vi "SET_SHUNT_n.vi"(2 "execute":bool, 7 "SHUNT values":cdb[](array[numeric]), 11 "error in (no error)":errorcluster) -> (4 "function return":string, 15 "error out":errorcluster)   [LabVIEW 2017, in "ZBOX_IS.lvlib"]
uses:
  ZBOX_IS.lvlib
panel:
  out "BytePtr":u8[](array[numeric])
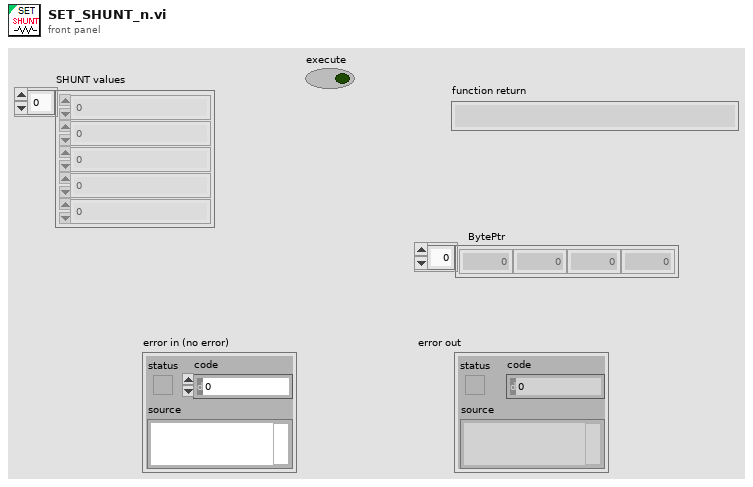
[diagram p1: front panel]
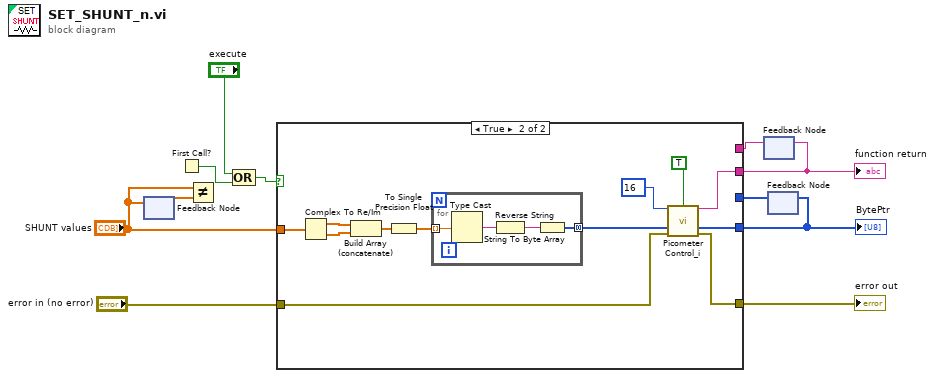
[diagram p0: block diagram]
diagram:
  n1 = feedback-in #1("SHUNT values") -> ()
  n2 = feedback #1() -> (w5:cdb[])  [unwired: 1 in]
  n3 = First Call?() -> (First Call?: T/F=w2:bool)
  n4 = Not Equal?(x="SHUNT values", y=w5) -> ()  [unwired: 1 out]
  n5 = Compound Arithmetic op=OR("execute", w2) -> (w3:bool)
  n6 = feedback #2() -> (w8:string)  [unwired: 1 in]
  n7 = feedback #3() -> (w6:u8[])  [unwired: 1 in]
  n8 = case shown="True" w3 {
    tunnel: "error in (no error)" -> [w14 w25]
    tunnel: [w14 w24] -> w10
    tunnel: [w13 w23] -> w9
    tunnel: "SHUNT values" -> [_ w17]
    tunnel: [w12 w16] -> w7
    tunnel: w8 -> [w13 _]
    tunnel: w6 -> [w12 _]
    frame False {
    }
    frame True {
      n9 = Complex To Re/Im(x + iy=w17) -> (x=w22:dbl[], y=w21:dbl[])
      n10 = Build Array (concatenate)(w22, w21) -> (w20:dbl[])
      n11 = To Single Precision Float(number=w20) -> (single precision float=w19:sgl[])
      n12 = for {
        tunnel: w19 -> [w30] mode=indexing
        tunnel: [w28] -> w18 mode=concatenating
        n13 = Type Cast(x=w30) -> (*(type *) &x=w27:string)  [unwired: 1 in]
        n14 = Reverse String(1:w27) -> (0:w29:string)
        n15 = String To Byte Array(string=w29) -> (unsigned byte array=w28:u8[])
      }
      n16 = call "Picometer Control_i.vi"("Cmd"=u8 16, "execute"=TRUE, "BytePtr"=w18, "error in (no error)"=w25) -> ("function return"=w23:string, "BytePtr"=w16:u8[], "error out"=w24:errorcluster)  [unwired: 7 in, 2 out]
    }
  }
  "error out" <- w10
  "function return" <- w9
  "BytePtr" <- w7
  n17 = feedback-in #2(w9) -> ()
  n18 = feedback-in #3(w7) -> ()
